vi "Set Log.vi"(8 "error in (no error)":errorcluster, 10 "Log":refnum<class "Debug Log.lvclass">, 11 "Debugger in":refnum<class "Debugger.lvclass">) -> (0 "error out":errorcluster, 3 "Debugger out":refnum<class "Debugger.lvclass">)   [LabVIEW 2020, in "Debugger.lvclass"]
uses:
  Debugger.lvclass
  Debugger.lvclass/Debugger.ctl
  Debug Log/Debug Log.lvclass
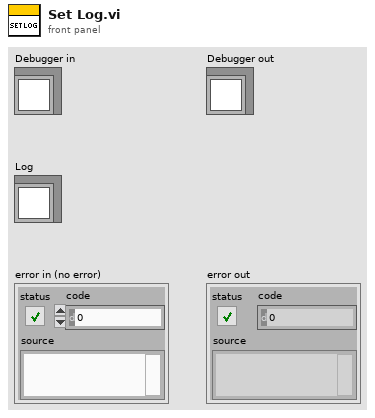
[diagram p1: front panel]
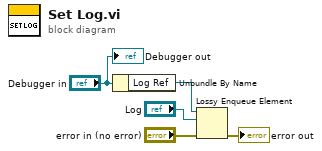
[diagram p0: block diagram]
diagram:
  n1 = Unbundle By Name("Debugger in") -> ("Log Ref"=w4:refnum<queue>)
  n2 = Lossy Enqueue Element(queue=w4, element="Log", error in (no error)="error in (no error)") -> (error out=→"error out":errorcluster)  [unwired: 3 out]
  "Debugger out" <- "Debugger in"
